vi "Save3DStack.vi"(0 "Experiment Name":string, 1 "Identify Name":string, 2 "3D Data":dbl[][][](array[numeric]), 3 "matrix_max":dbl, 4 "matrix_min":dbl, 5 "error in":errorcluster, 6 "File Name":string, 7 "Index Name":string, 8 "path":path, 10 "Specify Range?":bool=TRUE, 11 "Enable?":bool, 12 "Crop Pixels":u16=30, 13 "Time Stamp?":bool) -> (15 "img cancelled":bool, 19 "error out":errorcluster)   [LabVIEW 2015]
uses:
  ctiff.llb/__CTIFFNewFileAndStyleFLOAT32.vi
  ctiff.llb/__CTIFFAddNewPageFLOAT32.vi
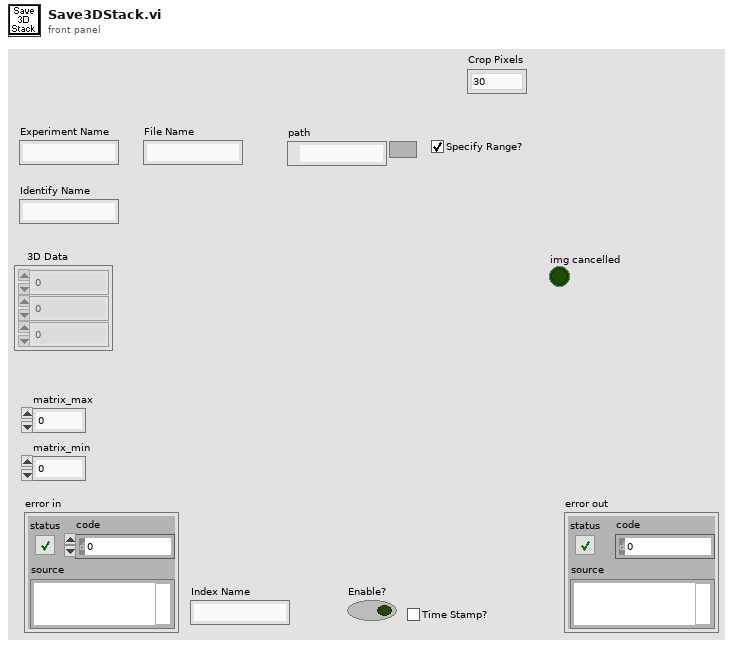
[diagram p1: front panel]
types:
  T1 = enum16{"open", "replace", "create", "open or create", "replace or create", "replace or create with confirmation"}
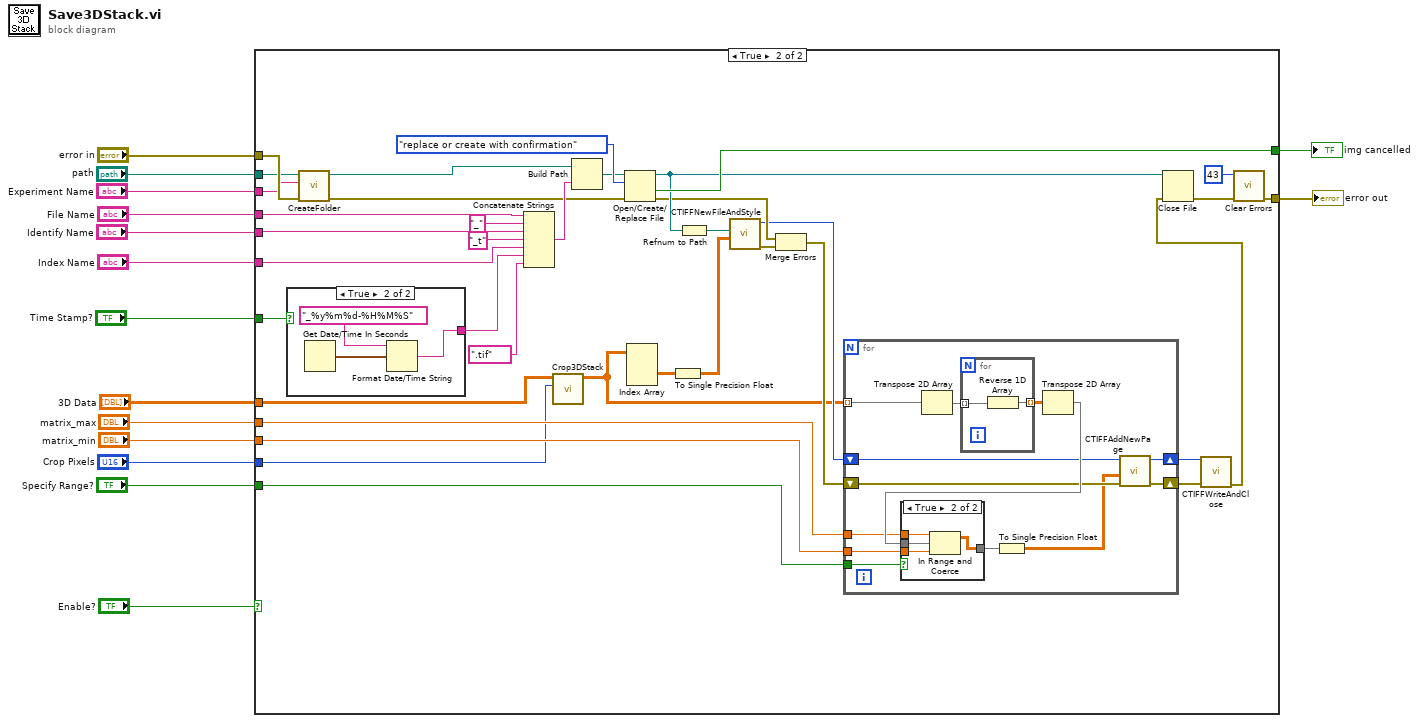
[diagram p0: block diagram]
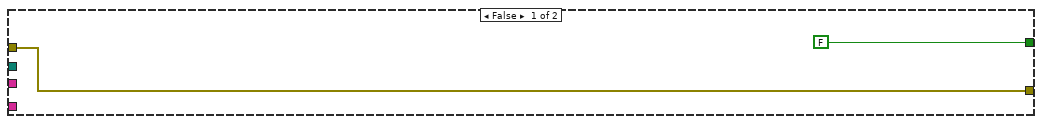
[diagram p2: hidden frame]
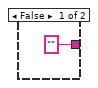
[diagram p4: hidden frame]
diagram:
  n1 = case shown="True" "Enable?" {
    tunnel: "error in" -> [w17 w54]
    tunnel: [w17 w39] -> w14
    tunnel: "Experiment Name" -> [_ w52]
    tunnel: "File Name" -> [_ w50]
    tunnel: "3D Data" -> [_ w20]
    tunnel: "path" -> [_ w53]
    tunnel: [FALSE ("save cancelled") w42] -> w6
    tunnel: "matrix_max" -> [_ w37]
    tunnel: "matrix_min" -> [_ w36]
    tunnel: "Identify Name" -> [_ w48]
    tunnel: "Time Stamp?" -> [_ w51]
    tunnel: "Specify Range?" -> [_ w35]
    tunnel: "Crop Pixels" -> [_ w19]
    tunnel: "Index Name" -> [_ w21]
    frame False {
    }
    frame True {
      n2 = case shown="True" w51 {
        tunnel: ["" w76] -> w23
        frame False {
        }
        frame True {
          n3 = Get Date/Time In Seconds() -> (seconds since 1Jan1904=w77:timestamp)
          n4 = Format Date/Time String(time format string (%c)="_%y%m%d-%H%M%S", seconds (now)=w77) -> (date/time string=w76:string)  [unwired: 1 in]
        }
      }
      n5 = call "CreateFolder.vi"("error in (no error)"=w54, "name"=w52, "base path"=w53) -> ("error out"=w45:errorcluster, "path out"=w46:path)  [unwired: 7 in]
      n6 = Concatenate Strings(w50, "_" ("string"), w48, "_t" ("string"), w21, w23, ".tif" ("string")) -> (w47:string)
      n7 = call "Crop3DStack.vi"("Crop Pixels"=w19, "3D Data"=w20) -> ("Cropped 3D Data"=w18:dbl[][][])  [unwired: 9 in]
      n8 = Build Path(base path=w46, name or relative path=w47) -> (appended path=w43:path)
      n9 = Open/Create/Replace File(file path (use dialog)=w43, error in=w45, operation (0:open)=T1."replace or create with confirmation") -> (refnum out=w38:refnum<file>, cancelled=w42:bool, error out=w33:errorcluster)  [unwired: 3 in]
      n10 = Index Array(array=w18) -> (element=w27:dbl[][])  [unwired: 3 in]
      n11 = To Single Precision Float(number=w27) -> (single precision float=w26:sgl[][])
      n12 = Refnum to Path(1:w38) -> (0:w34:path)
      n13 = call-poly "CTIFFNewFileAndStyle.vi"("image"=w26, "output_file"=w34) -> ("error"=w32:errorcluster, "CTIFF"=w25:i64)  [unwired: 8 in]
      n14 = Merge Errors(w33, w32) -> (w31:errorcluster)
      n15 = for {
        tunnel: w18 -> [w55] mode=indexing
        tunnel: w37 -> [w64]
        tunnel: w36 -> [w63]
        tunnel: w35 -> [w62]
        shift-right: [w60] -> w30
        shift-left: w31 -> [w61]
        shift-right: [w59] -> w29
        shift-left: w25 -> [w56]
        n16 = Transpose 2D Array(2D array=w55) -> (transposed array=w66:dbl[][])
        n17 = for {
          tunnel: w66 -> [w74] mode=indexing
          tunnel: [w73] -> w67 mode=indexing
          n18 = Reverse 1D Array(array=w74) -> (reversed array=w73:dbl[])
        }
        n19 = Transpose 2D Array(2D array=w67) -> (transposed array=w65:dbl[][])
        n20 = case shown="True" w62 {
          tunnel: w65 -> [w68 w72]
          tunnel: [w68 w71] -> w58
          tunnel: w64 -> [_ w70]
          tunnel: w63 -> [_ w69]
          frame False {
          }
          frame True {
            n21 = In Range and Coerce(upper limit=w70, x=w72, lower limit=w69) -> (coerced(x)=w71:dbl[][])  [unwired: 1 out]
          }
        }
        n22 = To Single Precision Float(number=w58) -> (single precision float=w57:sgl[][])
        n23 = call-poly "CTIFFAddNewPage.vi"("error"=w61, "image"=w57, "CTIFF"=w56) -> ("error"=w60:errorcluster, "CTIFF"=w59:i64)  [unwired: 7 in]
      }
      n24 = call "CTIFFWriteAndClose.vi"("error"=w30, "CTIFF"=w29) -> ("error"=w28:errorcluster)  [unwired: 9 in]
      n25 = Close File(refnum=w38, error in=w28) -> (error out=w40:errorcluster)  [unwired: 1 out]
      n26 = call <vilib>:"Clear Errors.vi"("error in (no error)"=w40, "specific error code to clear (0: all)"=43) -> ("error out"=w39:errorcluster)  [unwired: 4 in, 1 out]
    }
  }
  "error out" <- w14
  "img cancelled" <- w6
